vi "Log File Header Write.vi"(8 "error in":errorcluster, 10 "Raw Data Period":dbl=0.0001024, 11 "FPGA Refnum":T1) -> (0 "error out":errorcluster, 1 "offset for # rows":i64, 2 "concatenated string":string, 3 "Byte Stream File out":refnum<file>)   [LabVIEW 2018]
doc: "Author: Scott Hannahs <sth@magnet.fsu.edu>\nCopyright 2018 Florida State University, All rights reserved."
uses:
  RT Controls/FPGA SCH Digitizer Ref.ctl
  RT Host Globals.vi
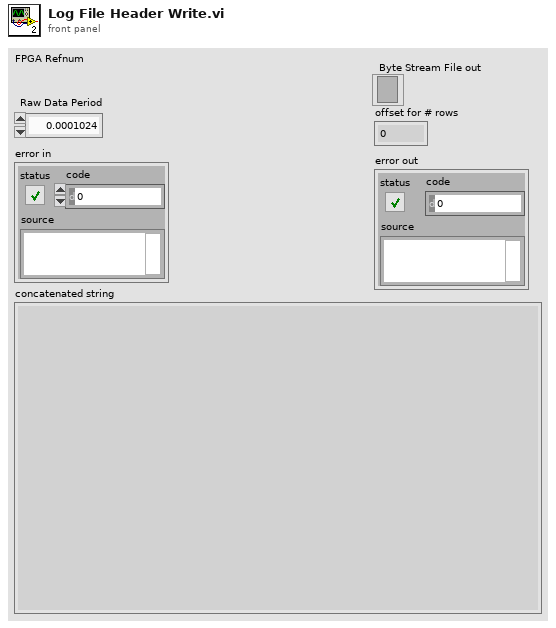
[diagram p1: front panel]
types:
  T1 = typedef "FPGA SCH Digitizer Ref.ctl" = refnum<k20>
  T2 = enum16{"open", "replace", "create", "open or create", "replace or create", "replace or create with confirmation"}
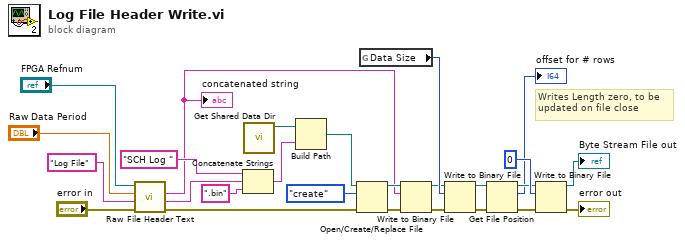
[diagram p0: block diagram]
diagram:
  # "Writes Length zero, to be \nupdated on file close"
  n1 = call "Raw File Header Text.vi"("error in (no error)"="error in", "Type"="Log File", "Raw Data Period"="Raw Data Period", "FPGA Refnum out"="FPGA Refnum") -> ("error out"=w13:errorcluster, "Date String"=w16:string, "concatenated string"=w15:string)  [unwired: 5 in]
  "concatenated string" <- w15
  n2 = Concatenate Strings("SCH Log " ("string"), w16, ".bin" ("string")) -> (w23:string)
  n3 = call "Get Shared Data Dir.vi"() -> ("Data Directory Path"=w26:path)  [unwired: 2 in, 1 out]
  n4 = Build Path(base path=w26, name or relative path=w23) -> (appended path=w22:path)
  n5 = Open/Create/Replace File(file path (use dialog)=w22, error in=w13, operation (0:open)=T2."create") -> (refnum out=w21:refnum<file>, error out=w20:errorcluster)  [unwired: 3 in, 1 out]
  n6 = global read "RT Host Globals.vi" "Data Size"() -> (w11:u32)
  n7 = Write to Binary File(file (use dialog)=w21, data=w15, error in=w20) -> (refnum out=w7:refnum<file>, error out=w8:errorcluster)  [unwired: 3 in, 1 out]
  n8 = Write to Binary File(file (use dialog)=w7, data=w11, error in=w8) -> (refnum out=w5:refnum<file>, error out=w2:errorcluster)  [unwired: 3 in, 1 out]
  n9 = Get File Position(4:w2, 7:w5) -> (0:w3:errorcluster, 2:→"offset for # rows":i64, 3:w4:refnum<file>)
  n10 = Write to Binary File(file (use dialog)=w4, data=u32 0 ("Data Size"), error in=w3) -> (refnum out=→"Byte Stream File out":refnum<file>, error out=→"error out":errorcluster)  [unwired: 3 in, 1 out]
